vi "Dequeue.vi"(8 "ErrorArray In":errorcluster[](array[cluster])) -> (0 "ErrorArray Out":errorcluster[](array[cluster]), 1 "Data":variant, 2 "Msg":string)   [LabVIEW 2014, in "TestFramework.lvlib"]
uses:
  TestFramework.lvlib
  TypeDef/MsgQueue.ctl
  <userlib>/NIST/NISTErrorLib/NISTErrorLib.lvlib
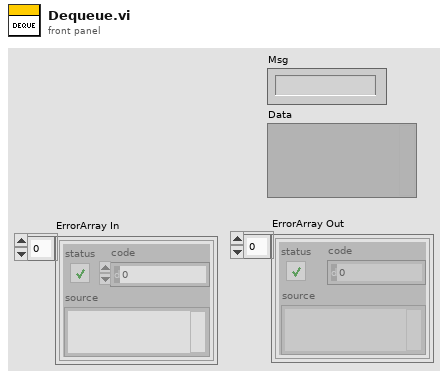
[diagram p1: front panel]
types:
  T1 = typedef "TestFramework.lvlib/MsgQueue.ctl" = cluster{"Msg":string, "Data":variant}
  T2 = typedef "TestFramework.lvlib/QueRef.ctl" = refnum<queue>
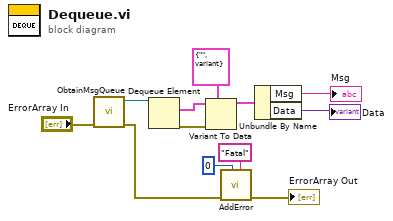
[diagram p0: block diagram]
diagram:
  n1 = call "ObtainMsgQueue.vi"("ErrorArray In"="ErrorArray In") -> ("ErrorArray Out"=w10:errorcluster[], "QueRef"=w11:T2)  [unwired: 9 in]
  n2 = Dequeue Element(queue=w11) -> (element=w6:T1, error out=w5:errorcluster)  [unwired: 2 in, 2 out]
  n3 = Variant To Data(error in=w5, type=T1 {"Msg"="", "Data"=variant} ("MsgQueue"), Variant=w6) -> (data=w3:T1)  [unwired: 1 out]
  n4 = call <userlib>:"AddError.vi"("Severity"="Fatal" ("String"), "Priority"=u8 0, "ErrorArray"=w10) -> ("ErrorArray"=→"ErrorArray Out":errorcluster[])  [unwired: 7 in, 1 out]
  n5 = Unbundle By Name(w3) -> ("Msg"=→"Msg":string, "Data"=→"Data":variant)
